vi "GT Get Profile Scale.vi"(7 "pBeta":i32, 8 "error in (no error)":errorcluster caption="错误输入（无错误）", 9 "pAlpha":i32, 10 "axis":i16, 11 "cardNum":i16) -> (0 "error out":errorcluster caption="错误输出", 1 "pAlpha out":i32, 3 "function return":i16, 5 "pBeta out":i32)   [LabVIEW 2014, in "gts.lvlib"]
doc: "GT_API GT_GetProfileScale(short cardNum,short axis,long *pAlpha,long *pBeta);"
uses:
  gts.lvlib
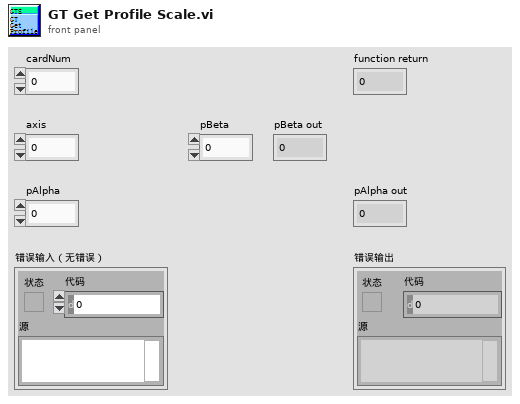
[diagram p1: front panel]
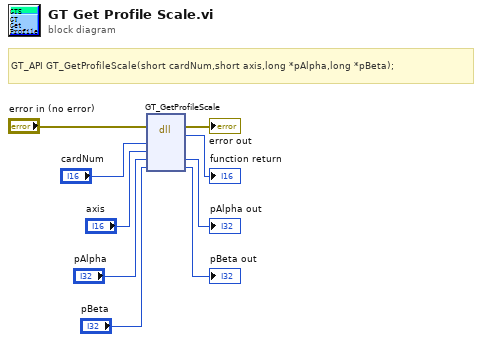
[diagram p0: block diagram]
diagram:
  # "GT_API GT_GetProfileScale(short cardNum,short axis,long *pAlpha,long *pBeta);"
  n1 = dll-call lib="PTH2habs D固高科技资料GTS控制卡GTS卡18年上半年资料dllVC32bit\nmulti_cardgts.*" fn="GT_GetProfileScale"(error in="error in (no error)", "cardNum"="cardNum", "axis"="axis", "pAlpha"="pAlpha", "pBeta"="pBeta") -> (error out=→"error out":errorcluster, →"function return":i16, "pAlpha"=→"pAlpha out":i32, "pBeta"=→"pBeta out":i32)  [unwired: 4 in, 1 out]
